vi "RP Lockin Proccess.vi"(4 "Save output":bool, 6 "Filter type":enum16{"None", "IIR", "FIR"}(ring)=enum."IIR", 8 "Error In":errorcluster, 9 "X channel":string, 10 "Configuration":T1={"Time constant"=0.0, "Phase"=0.0, "Signal channels"=[], "Group"="p", "Clip units of Ts off"=1.0, "X channel"=""} {"Phase" scale=-180.0..180.0; "Time constant" format="%#_6ps"}, 11 "Signal file":path) -> (0 "Error Out":errorcluster)   [LabVIEW 2015]
uses:
  Measure_extentions/Post-Processors/Lockin Processor/Lockin Processor Configuration.ctl
panel:
  in  "CH index":i32
  in  "X tiime shift":dbl format="%#_6p"
  out "Phase":dbl
  out "Waveform Graph 2":waveform(dbl)(graph)
  in  "Fix time delay":bool=TRUE
  out "XY Graph":cluster{dbl[], "Y":dbl[]}[](graph)
  out "Waveform Graph":waveform(dbl)[](graph)
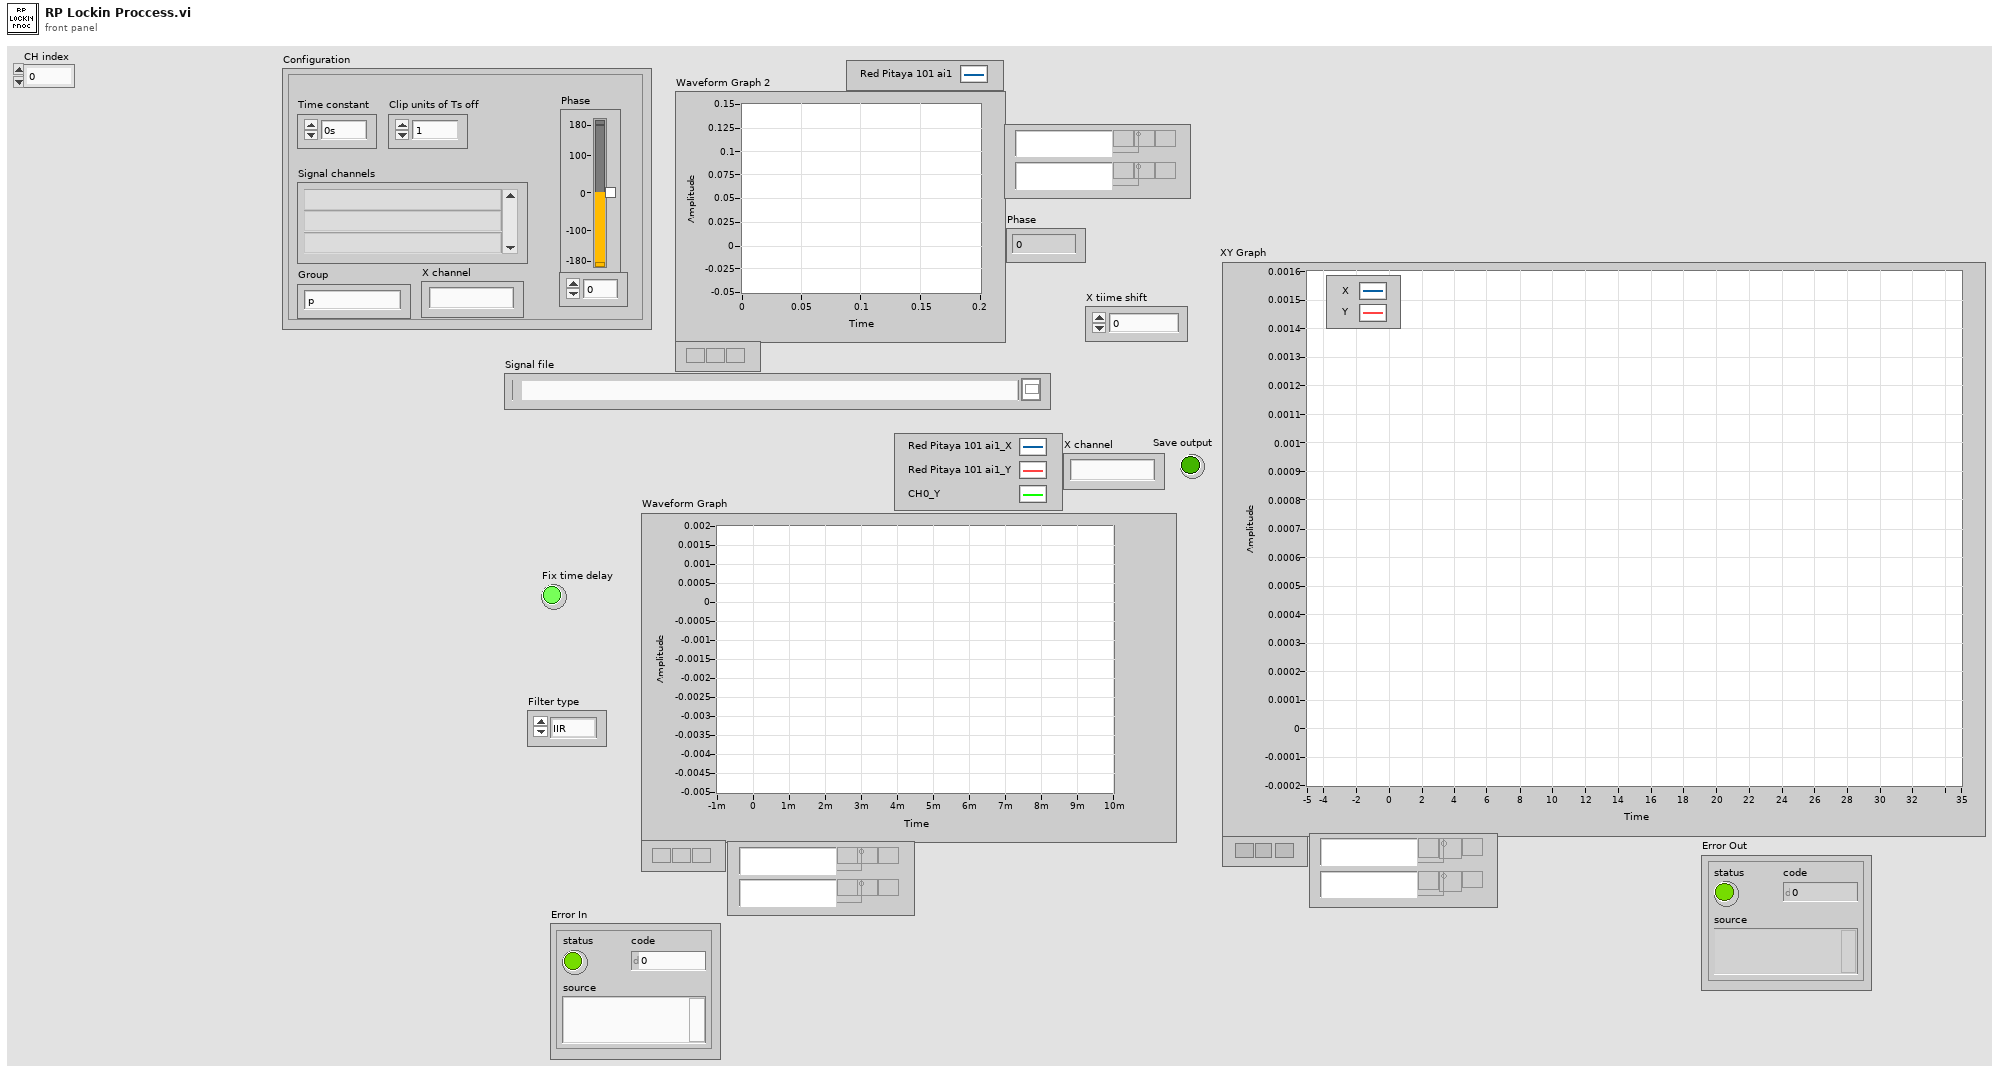
[diagram p1: front panel]
types:
  T1 = typedef "Lockin Processor Configuration.ctl" = cluster{"Time constant":dbl, "Phase":dbl, "Signal channels":string[], "Group":string, "Clip units of Ts off":dbl, "X channel":string}
  T2 = enum16{"open", "open or create", "create or replace", "create", "open (read-only)"}
  T3 = cluster{"Waveform":waveform(dbl), "Waveform":waveform(dbl)}
  T4 = cluster{"Waveform":waveform(dbl), "Waveform":waveform(dbl)}[]
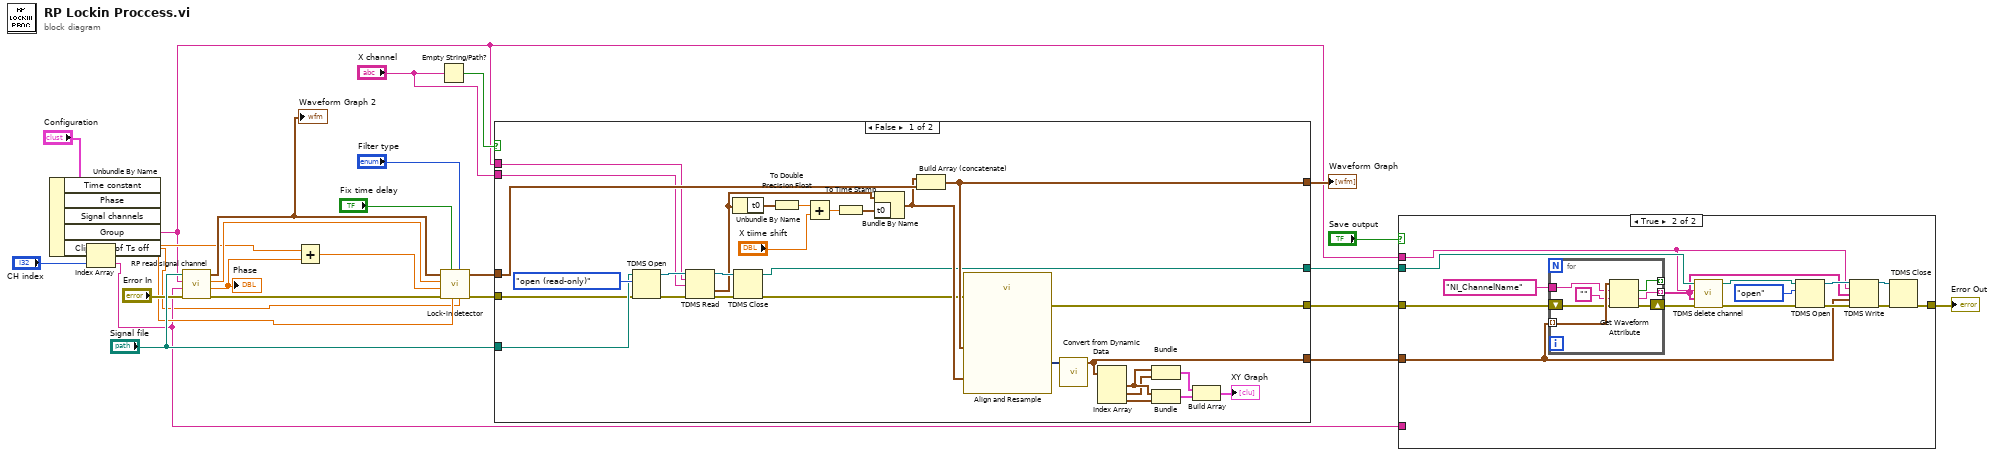
[diagram p0: block diagram]
diagram:
  n1 = Unbundle By Name("Configuration") -> ("Time constant"=w7:dbl, "Phase"=w6:dbl, "Signal channels"=w5:string[], "Group"=w2:string, "Clip units of Ts off"=w1:dbl)
  n2 = Index Array(array=w5, index="CH index") -> (element=w3:string)
  n3 = call "RP read signal channel.vi"("Error In"="Error In", "Channel name"=w3, "group name in"=w2, "File Path Control"="Signal file") -> ("Error Out"=w25:errorcluster, "Phase"=w26:dbl, "Frequency"=w27:dbl, "Data out"=w13:waveform(dbl))  [unwired: 2 in, 2 out]
  "Waveform Graph 2" <- w13
  "Phase" <- w26
  n4 = Add(x=w6, y=w26) -> (x+y=w21:dbl)
  n5 = Empty String/Path?(string/path="X channel") -> (empty?=w12:bool)
  n6 = call "Lock-in detector.vi"("Clip units of Ts off"=w1, "Filter type"="Filter type", "Time constant"=w7, "Fix time delay"="Fix time delay", "Error In"=w25, "Phase"=w21, "Frequency"=w27, "Data in"=w13) -> ("Error Out"=w15:errorcluster, "Data out"=w23:waveform(dbl)[])  [unwired: 2 in]
  n7 = case shown="False" w12 {
    tunnel: w23 -> [w51 w59]
    tunnel: [w44 w59] -> w22
    tunnel: [w43 w58] -> w19
    tunnel: [w40 w59] -> w17
    tunnel: "Signal file" -> [w39 w58]
    tunnel: w15 -> [w36 w57]
    tunnel: [w37 w57] -> w14
    tunnel: "X channel" -> [w29 _]
    tunnel: w2 -> [w28 _]
    frame False {
      n8 = TDMS Open(8:w36, 10:T2."open (read-only)" ("operation (0:open)"), 11:w39) -> (0:w55:errorcluster, 3:w54:refnum<k34>)  [unwired: 4 in]
      n9 = TDMS Read(0:w54, 5:w28, 7:w29, 11:w55) -> (4:w52:refnum<k34>, 10:w30:waveform(dbl), 15:w53:errorcluster)  [unwired: 4 in, 3 out]
      n10 = Unbundle By Name(w30) -> ("t0"=w35:timestamp)
      n11 = TDMS Close(8:w53, 11:w52) -> (0:w38:errorcluster, 3:w43:path)
      n12 = To Double Precision Float(number=w35) -> (double precision float=w34:dbl)
      n13 = Add(x=w34, y="X tiime shift") -> (x+y=w32:dbl)
      n14 = To Time Stamp(1:w32) -> (0:w31:timestamp)
      n15 = Bundle By Name(cluster=w30, "t0"=w31) -> (w50:waveform(dbl))
      n16 = Build Array (concatenate)(w50, w51) -> (w44:waveform(dbl)[])
      n17 = call "Align and Resample"("Reference Signal"=w50, "error in (no error)"=w38, "Signals"=w44) -> ("error out"=w37:errorcluster, "Resampled Signals"=w49:dynamicdata)  [unwired: 6 in, 1 out]
      n18 = call "Convert from Dynamic Data"("Dynamic Data Type"=w49) -> ("Array of Waveform"=w40:waveform(dbl)[])  [unwired: 3 in]
      n19 = Index Array(array=w40) -> (element #1=w48:waveform(dbl), element #2=w42:waveform(dbl), element #3=w41:waveform(dbl))  [unwired: 3 in]
      n20 = Bundle("Waveform"=w48, "Waveform"=w42) -> (w47:T3)  [unwired: 1 in]
      n21 = Bundle("Waveform"=w48, "Waveform"=w41) -> (w46:T3)  [unwired: 1 in]
      n22 = Build Array(w47, w46) -> (→"XY Graph":T4)
    }
    frame True {
    }
  }
  "Waveform Graph" <- w22
  n23 = case shown="True" "Save output" {
    tunnel: w19 -> [_ w71]
    tunnel: w14 -> [w60 w65]
    tunnel: [w60 w73] -> w18
    tunnel: w3 -> [_ _]
    tunnel: w17 -> [_ w63]
    tunnel: w2 -> [_ w62]
    frame False {
    }
    frame True {
      n24 = for {
        tunnel: w63 -> [w82] mode=indexing
        tunnel: "NI_ChannelName" ("name") -> [w81]
        tunnel: [w80] -> _ mode=indexing
        tunnel: [w76] -> w61 mode=indexing
        shift-right: [w78] -> w64
        shift-left: w65 -> [w79]
        n25 = Get Waveform Attribute(4:w79, 5:"", 6:w81, 7:w82) -> (0:w78:errorcluster, 1:w76:string, 2:w80:bool)  [unwired: 1 out]
      }
      n26 = call "TDMS delete channel.vi"("error in (no error)"=w64, "Channels"=w61, "group name"=w62, "file path"=w71) -> ("error out"=w70:errorcluster, "file path out"=w69:path)  [unwired: 5 in, 1 out]
      n27 = TDMS Open(8:w70, 10:T2."open" ("operation (0:open)"), 11:w69) -> (0:w67:errorcluster, 3:w68:refnum<k34>)  [unwired: 4 in]
      n28 = TDMS Write(0:w68, 5:w62, 7:w61, 9:w63, 11:w67) -> (4:w75:refnum<k34>, 15:w74:errorcluster)  [unwired: 1 in, 2 out]
      n29 = TDMS Close(8:w74, 11:w75) -> (0:w73:errorcluster)  [unwired: 1 out]
    }
  }
  "Error Out" <- w18
